vi "Data_Packets_To_Transmitter_Table_Formatter.vi"(8 "error in (no error)":errorcluster, 11 "Data Packets In":T1[](array[typedef])) -> (0 "error out":errorcluster, 3 "Table contents":string[][](array[string]))   [LabVIEW 2017]
uses:
  Controls/Data Packets/Data_Packet.ctl
  Controls/Packet/Packet.ctl
  Controls/Packet/Packet_Direction.ctl
  Controls/Packet/Packet_Type.ctl
  Controls/Packet/Packet_Priority.ctl
  Controls/Data Packets/Parameter.ctl
  Controls/Data Packets/Parameter_Data_Type.ctl
  Controls/Data Packets/Data_Packet_Transmit_Mode.ctl
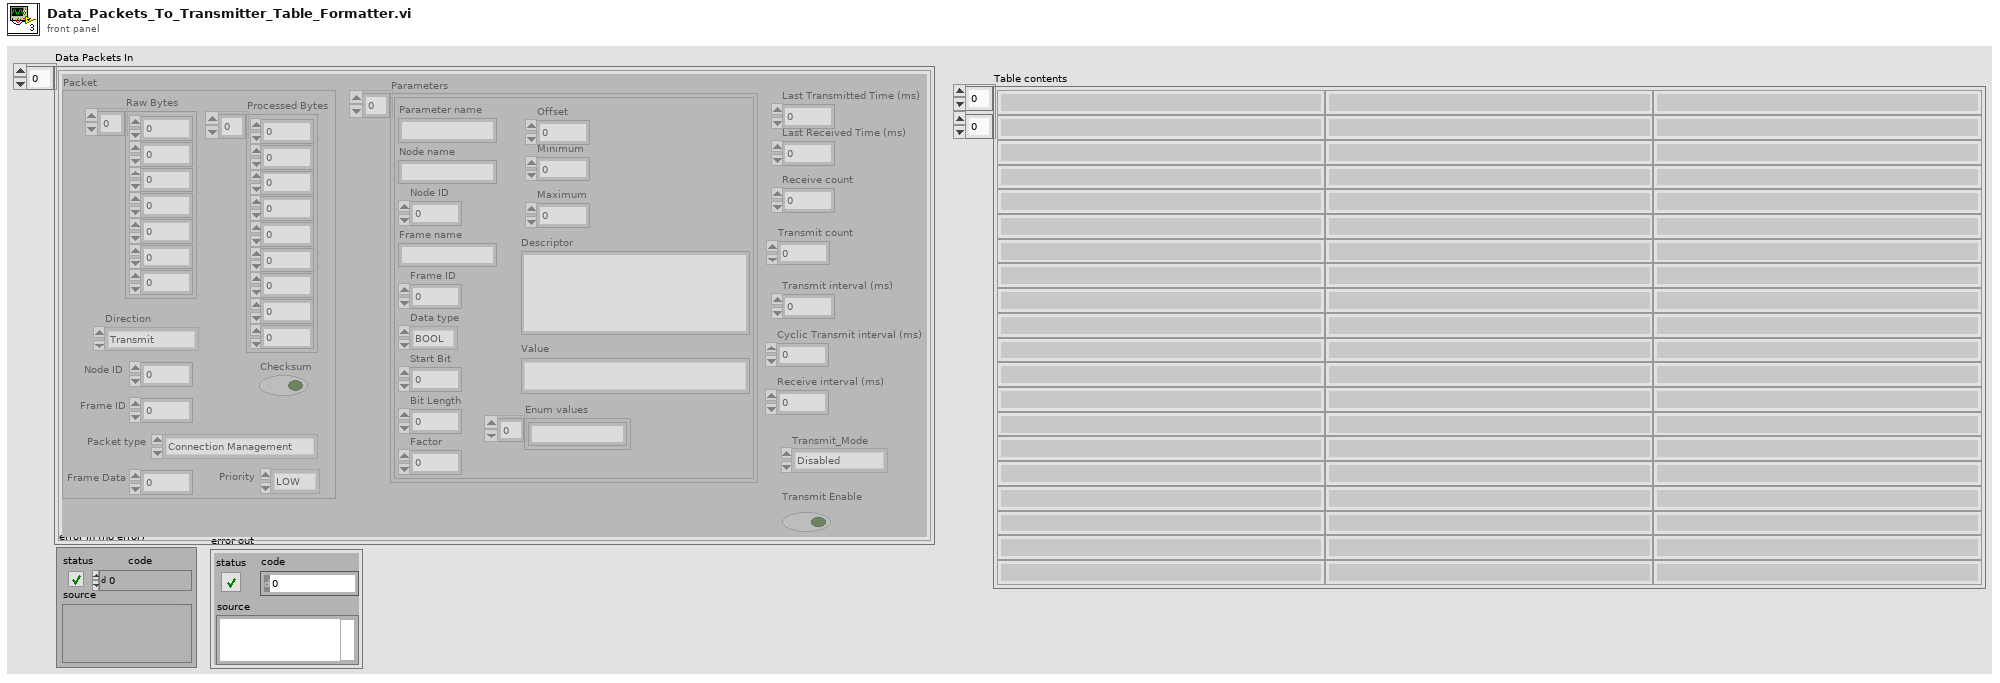
[diagram p1: front panel]
types:
  T1 = typedef "Data_Packet.ctl" = cluster{"Packet":T2, "Parameters":T6[], "Last Received Time (ms)":u64, "Receive count":i32, "Transmit count":i32, "Transmit interval (ms)":u32, "Last Transmitted Time (ms)":u64, "Receive interval (ms)":u32, "Transmit_Mode":T8, "Transmit Enable":bool, "Cyclic Transmit interval (ms)":u32}
  T2 = typedef "Packet.ctl" = cluster{"Raw Bytes":u8[], "Checksum":bool, "Direction":T3, "Processed Bytes":u8[], "Node ID":u8, "Packet type":T4, "Frame Data":u32, "Priority":T5, "Frame ID":u8}
  T3 = typedef "Packet_Direction.ctl" = enum16{"Transmit", "Receive", "Bidirectional"}
  T4 = typedef "Packet_Type.ctl" = enum16{"Data", "Connection Management", "Remote Request", "Error/Status"}
  T5 = typedef "Packet_Priority.ctl" = enum16{"LOW", "HIGH"}
  T6 = typedef "Parameter.ctl" = cluster{"Parameter name":string, "Node name":string, "Node ID":u8, "Frame name":string, "Frame ID":u8, "Data type":T7, "Start Bit":i32, "Bit Length":i32, "Factor":dbl, "Offset":dbl, "Minimum":dbl, "Maximum":dbl, "Descriptor":string, "Enum values":string[], "Value":string}
  T7 = typedef "Parameter_Data_Type.ctl" = enum16{"BOOL", "UNSIGNED", "SIGNED", "FLOAT32", "ENUM"}
  T8 = typedef "Data_Packet_Transmit_Mode.ctl" = enum16{"Disabled", "Single", "Cyclic"}
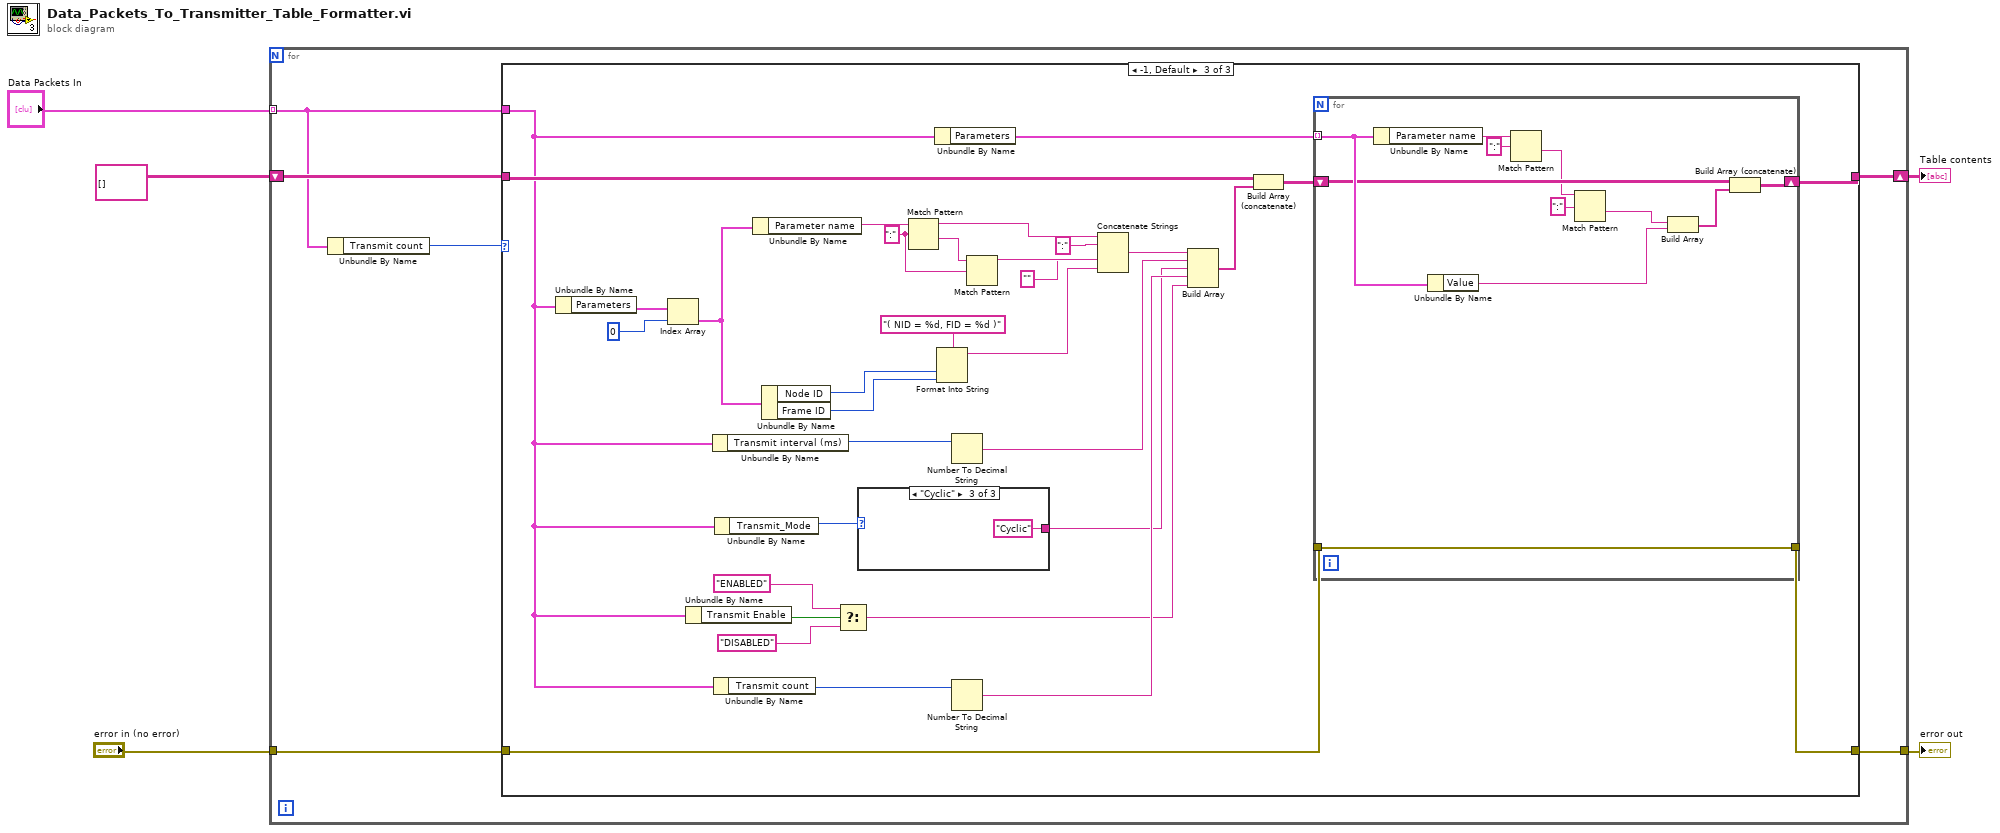
[diagram p0: block diagram]
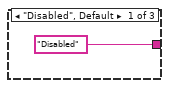
[diagram p4: hidden frame]
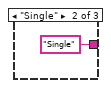
[diagram p5: hidden frame]
diagram:
  n1 = for {
    tunnel: "Data Packets In" -> [w7] mode=indexing
    tunnel: "error in (no error)" -> [w11]
    tunnel: [w10] -> w2
    shift-right: [w8] -> w3
    shift-left: string[][] [] -> [w9]
    n2 = Unbundle By Name(w7) -> ("Transmit count"=w6:i32)
    n3 = case shown="-1, Default" w6 {
      tunnel: w11 -> [w13 w15 w25]
      tunnel: [w13 w15 w24] -> w10
      tunnel: w9 -> [w12 w14 w30]
      tunnel: [w12 w14 w27] -> w8
      tunnel: w7 -> [_ _ w20]
      frame -2 {
      }
      frame 0 {
      }
      frame -1, Default {
        w44 = ":" ("regular expression")
        n4 = Unbundle By Name(w20) -> ("Parameters"=w48:T6[])
        n5 = Index Array(array=w48, index=0) -> (element=w34:T6)
        n6 = Unbundle By Name(w20) -> ("Transmit Enable"=w19:bool)
        n7 = Unbundle By Name(w20) -> ("Transmit interval (ms)"=w33:u32)
        n8 = Unbundle By Name(w20) -> ("Transmit count"=w31:i32)
        n9 = Unbundle By Name(w20) -> ("Transmit_Mode"=w22:T8)
        n10 = Unbundle By Name(w34) -> ("Parameter name"=w46:string)
        n11 = Unbundle By Name(w34) -> ("Node ID"=w37:u8, "Frame ID"=w36:u8)
        n12 = Select(t="ENABLED", s=w19, f="DISABLED") -> (s? t:f=w16:string)
        n13 = case shown="\"Cyclic\"" w22 {
          tunnel: ["Disabled" "Single" "Cyclic"] -> w21
          frame "Disabled", Default {
          }
          frame "Single" {
          }
          frame "Cyclic" {
          }
        }
        n14 = Match Pattern(string=w46, regular expression=w44) -> (before substring=w43:string, after substring=w45:string)  [unwired: 1 in, 2 out]
        n15 = Unbundle By Name(w20) -> ("Parameters"=w26:T6[])
        n16 = Format Into String(format string="( NID = %d, FID = %d )", w37, w36) -> (resulting string=w35:string)  [unwired: 2 in, 1 out]
        n17 = Number To Decimal String(number=w33) -> (decimal integer string=w32:string)  [unwired: 1 in]
        n18 = Number To Decimal String(number=w31) -> (decimal integer string=w23:string)  [unwired: 1 in]
        n19 = Match Pattern(string=w45, regular expression=w44) -> (before substring=w41:string)  [unwired: 1 in, 3 out]
        n20 = Concatenate Strings(w43, ":" ("string"), w41, "" ("string"), w35) -> (w40:string)
        n21 = Build Array(w40, w32, w21, w23, w16) -> (w29:string[])
        n22 = Build Array (concatenate)(w30, w29) -> (w28:string[][])
        n23 = for {
          shift-right: [w55] -> w27
          shift-left: w28 -> [w57]
          tunnel: w26 -> [w58] mode=indexing
          tunnel: w25 -> [w54]
          tunnel: [w54] -> w24
          n24 = Unbundle By Name(w58) -> ("Parameter name"=w62:string)
          n25 = Unbundle By Name(w58) -> ("Value"=w52:string)
          n26 = Match Pattern(string=w62, regular expression=":") -> (after substring=w53:string)  [unwired: 1 in, 3 out]
          n27 = Match Pattern(string=w53, regular expression=":") -> (after substring=w59:string)  [unwired: 1 in, 3 out]
          n28 = Build Array(w59, w52) -> (w56:string[])
          n29 = Build Array (concatenate)(w57, w56) -> (w55:string[][])
        }
      }
    }
  }
  "Table contents" <- w3
  "error out" <- w2
